vi "UID Already Exists--error.vi"() -> (2 "Error":errorcluster)   [LabVIEW 2025, in "jettl.lvlib" / "Error.lvlib"]
uses:
  Error.lvlib
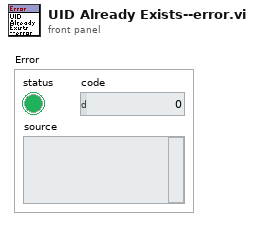
[diagram p1: front panel]
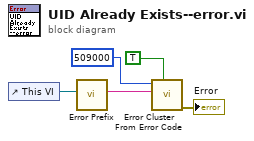
[diagram p0: block diagram]
diagram:
  n1 = control-ref of="This VI"() -> (w2:refnum<vi>)
  n2 = call "Error Prefix.vi"("VI Ref"=w2) -> ("Prefix"=w1:string)  [unwired: 10 in]
  n3 = call <vilib>:"Error Cluster From Error Code.vi"("show call chain? (False)"=TRUE, "error message (\"\")"=w1, "error code (0)"=509000) -> ("error out"=→"Error":errorcluster)  [unwired: 6 in]
